vi "MSScript_Calc_Round.vi"(6 "Value Error?":bool[](array[boolean]), 8 "ArrayVariable in":ext[](array[numeric]), 9 "Param Items":i32) -> (0 "ArrayVariable out":ext[](array[numeric]), 2 "CmdError?":bool)   [LabVIEW 2018, in "MSScript.lvclass"]
uses:
  MSScript.lvclass
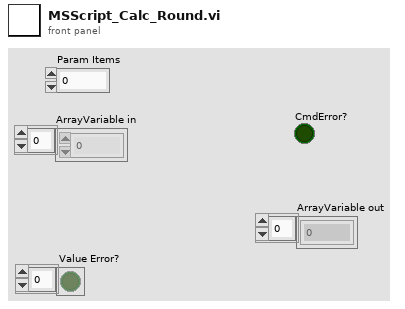
[diagram p1: front panel]
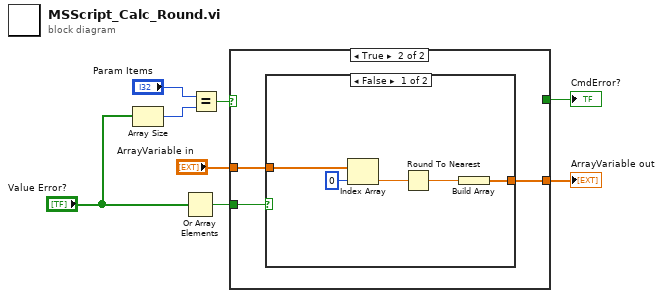
[diagram p0: block diagram]
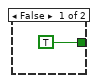
[diagram p2: hidden frame]
diagram:
  n1 = Array Size(array="Value Error?") -> (size(s)=w4:i32)
  n2 = Or Array Elements(Boolean array="Value Error?") -> (logical OR=w6:bool)
  n3 = Equal?(x="Param Items", y=w4) -> (x = y?=w2:bool)
  n4 = case shown="True" w2 {
    tunnel: [TRUE _] -> w1
    tunnel: w6 -> [_ w12]
    tunnel: "ArrayVariable in" -> [_ w11]
    tunnel: [_ w10] -> w8
    frame False {
    }
    frame True {
      n5 = case shown="False" w12 {
        tunnel: w11 -> [w16 _]
        tunnel: [w15 _] -> w10
        frame False {
          n6 = Index Array(array=w16, index=0) -> (element=w14:ext)
          n7 = Round To Nearest(number=w14) -> (nearest integer value=w13:ext)
          n8 = Build Array(w13) -> (w15:ext[])
        }
        frame True {
        }
      }
    }
  }
  "ArrayVariable out" <- w8
  "CmdError?" <- w1
